vi "Save bline to memory2.vi"(0 "PSOCTSpectral Bline":u16[](array[numeric]), 1 "action":T1=enum."Save(ThorOCT)", 5 "index (row)":i32, 9 "PSOCT Spatial Bline":sgl[](array[numeric]), 11 "error in":errorcluster) -> (15 "error out":errorcluster)   [LabVIEW 2018]
uses:
  Controls/Save Bline to Mem Control.ctl
  Controls/FGV Actions.ctl
  Controls/Queue Manager Actions.ctl
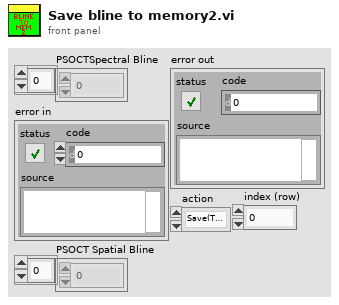
[diagram p1: front panel]
types:
  T1 = typedef "Save Bline to Mem Control.ctl" = enum16{"Output data", "Save(ThorOCT)", "Save(PSOCT)", "FFT and Save", "Uninit", "PSOCT Spectral buffer Set", "PSOCT Spatial buffer Set", "PSOCT Spectral buffer Init", "PSOCT Spatial buffer Init", "ThorOCT Spectral buffer Init", "ThorOCT Spatial buffer Init", "ThorOCT Spectral buffer Set", "ThorOCT Spatial buffer Set", "ThorOCT Spectral Save", "Alazar Spectral Save", "PSOCT save all"}
  T2 = typedef "FGV Actions.ctl" = enum16{"Init", "Set", "Get", "Clear"}
  T3 = typedef "System Parameters.ctl" = cluster{"Optical Parameters":T4, "Vibratome":T5, "Table Stages":T6, "Imaging Parameter":T9, "Galvo HW Parameters":cluster{"Analog Out Channel":tag, "Min Voltage":dbl, "Max Voltage":dbl, "Pixel Clock Source":tag, "Sample Rate":dbl, "Line Clock Out Ch":tag, "2P ready check":tag}, "Alazar parameters":T11, "Mosaic Paramter":cluster{"X Axis":cluster{"Start [mm]":dbl, "Steps [pts]":dbl, "End [mm]":dbl}, "Y Axis":cluster{"Start [mm]":dbl, "Steps [pts]":dbl, "End [mm]":dbl}, "Scan Pattern":enum16{"Uni-directional", "Bi-Directional", "Spiral Out", "Spiral In"}, "Overlap Options":cluster{"Overlap Type":enum16{"No Overlap", "X Only", "Y Only", "X and Y"}, "Percent Overlap":u8, "Justify":enum16{"Start", "Center", "End"}}}, "Manual Controls":T18, "Vibratome Axis":T21}
  T4 = typedef "Optical Parameters.ctl" = cluster{"Obj. Focal Length [mm]":dbl, "Scan Lens EFL[mm]":dbl, "Tube Lens EFL[mm]":dbl, "Galvo V Range (+/-)":dbl, "Galvo Max Half Angle [Deg]":dbl, "Max Galvo Range[%]":dbl}
  T5 = typedef "Vibratome Parameters.ctl" = cluster{"Z Bottom [mm]":dbl, "Pre Cut Dwell [s]":dbl, "Blade Frequency [RPM]":u16, "Slice Speed [mm/s]":dbl, "Post Cut Dwell [s]":dbl, "Ramp Time [s]":dbl, "Start X [mm]":dbl, "Start Y [mm]":dbl, "Slice Length [mm]":dbl, "Slice Axis":enum16{"X Axis", "Y Axis", "Z Axis"}, "Controller VISA Ref":refnum<visa-resource-name>, "Blade Frequency [Hz]":u16, "Analog Out Channel":tag, "Pixel Clock Source":tag}
  T6 = typedef "Translation Stage Parameters.ctl" = cluster{"X Stage":T7, "Y Stage":T7, "Z Stage":T7}
  T7 = typedef "Translation Stage Cluster.ctl" = cluster{"Position":dbl, "Is.Enabled?":bool, "Is.Connected?":bool, "Device SN":string, "AccelerationMaximum":dbl, "VelocityMaximum":dbl, "Acceleration":dbl, "Velocity":dbl, "waitTimeout (ms)":i32, "Model":T8, "Is.Homed?":bool, "MOVE":bool}
  T8 = typedef "Translation Stage Types.ctl" = enum16{"None", "Thorlabs LTS", "Thorlabs MLJ"}
  T9 = typedef "Imaging Parameters.ctl" = cluster{"Raster Scan Direction":T10, "Pixel Dwell Time [Clock Cycles]":u16, "Flyback Time [Clock Cycles]":u16, "XY Center [um]":cluster{"X":dbl, "Y":dbl}, "Pixel Step Size [um] X":dbl, "XY Image Size":enum16{"32 x 32", "64 x 64", "128 x 128", "256 x 256", "512 x 512", "1024 x 1024", "2048 x 2048"}, "Custom":bool, "Custom Size":cluster{"X":u16, "Y":u16}, "Line Averages":u8, "Pixel Step Size [um] Y":dbl}
  T10 = typedef "Scan Direction.ctl" = enum16{"Uni Directional", "Bi Directional", "None"}
  T11 = typedef "Alazar parameters.ctl" = cluster{"Trigger Settings":cluster{"General Trigger Settings":T12, "Trigger Engine 1":T13, "Trigger Engine 2":T13}, "Device ID":T14, "Ch A Input Control":T15, "Ch B Input Control":T15, "Acq Settings":T16, "Capture Clock":T17}
  T12 = typedef "General Trigger Settings.ctl" = cluster{"Trigger Operation":u32, "Coupling ID":u32, "Range ID":u32, "Delay":u32, "Timeout Ticks":u32, "Mode":u32, "Parameter":u32}
  T13 = typedef "Trigger Engine Controls.ctl" = cluster{"Trigger Engine":u32, "Source":u32, "Slope":u32, "Level":u32}
  T14 = typedef "Alazar Device ID.ctl" = cluster{"System ID":u32, "Board ID":u32}
  T15 = typedef "Channel Input Controls.ctl" = cluster{"Channel":u8, "Coupling":u32, "Range":u32, "Impedance":u32}
  T16 = typedef "Alazar Acquisition Settings.ctl" = cluster{"Record Length":u32, "Offset":u32, "Records Per Buffer":u32, "Records Count (Records/Acq)":u32, "Window Type":u32, "Footer":u32, "Samples per record":u32, "Output Format":u32}
  T17 = typedef "Clock Controls.ctl" = cluster{"Sample Rate":u32, "Decimation":u32, "Source":u32, "Edge":u32}
  T18 = typedef "Manual Controls.ctl" = cluster{"Z0":dbl, "First image height":dbl, "Data Path":path, "Save parameters":T19, "Center Galvos":bool, "Acquisition mode":T20, "PSOCT Channel":u32, "Save":bool, "AIP rotation angle":dbl, "ret ds":bool, "Pause?":bool, "Outgoing Mail Server (SMTP)":string, "Email":string, "Password":string, "Carrier 1":enum16{"T-Mobile", "AT&T", "Verizon", "Sprint"}, "phone number 1":string, "Subject":string, "Message":string, "blocker position":enum16{"every two slices", "Nat slices", "None"}, "Carrier 2":enum16{"T-Mobile", "AT&T", "Verizon", "Sprint"}, "phone number 2":string}
  T19 = typedef "FFT parameters.ctl" = cluster{"start pixel":i32, "#pixels to save":i32}
  T20 = typedef "FFT mode.ctl" = enum16{"ThorOCT B line", "ThorOCT Spectral", "ThorOCT FFT", "Alazar B line", "Alazar FFT", "GPU FFT", "Alazar Spectral", "Simulation", "auto adjust focus", "Save all"}
  T21 = typedef "Vibratome Param.ctl" = cluster{"Start [mm](first cut height)":dbl, "slice thickness[um]":dbl, "#slice":u16, "image thickness(um)":dbl, "#images":u16, "30um?":bool}
  T22 = typedef "Queue Manager Actions.ctl" = enum16{"Init", "Enqueue", "Enqueue All", "Preview Queue", "Dequeue", "Get Status", "Flush Queue", "Flush All Queues", "Release All Queues", "Release Queue", "Enqueue at Opposite End"}
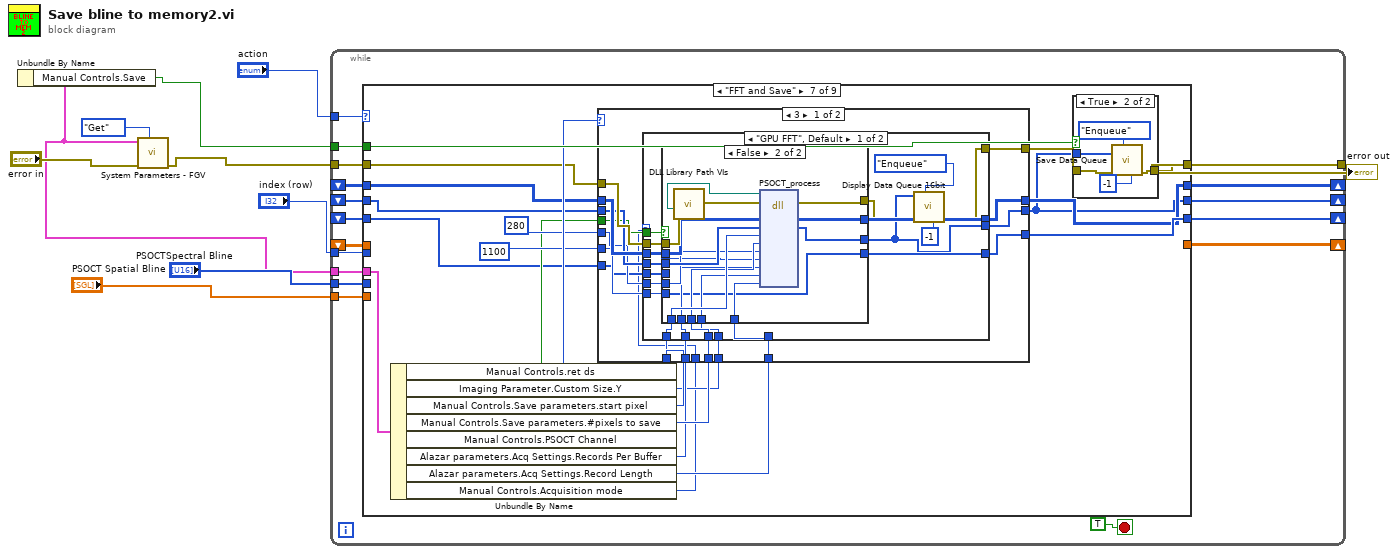
[diagram p0: block diagram]
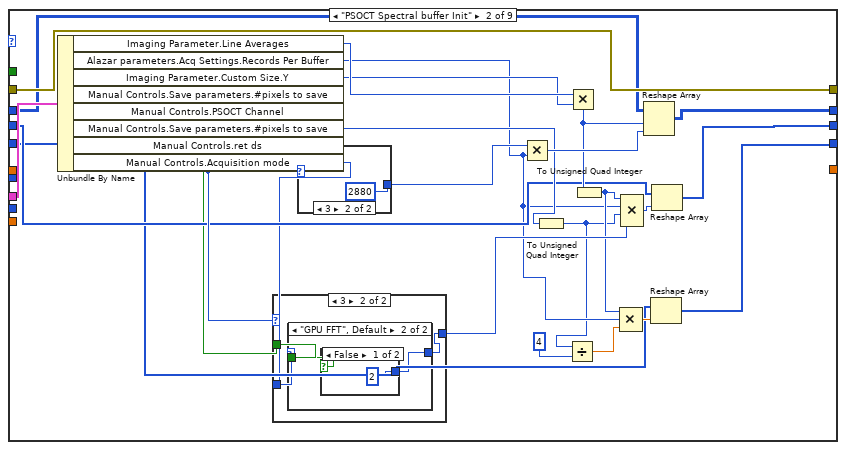
[diagram p3: hidden frame]
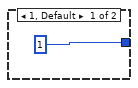
[diagram p4: hidden frame]
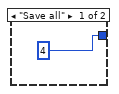
[diagram p5: hidden frame]
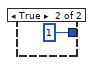
[diagram p6: hidden frame]
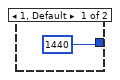
[diagram p7: hidden frame]
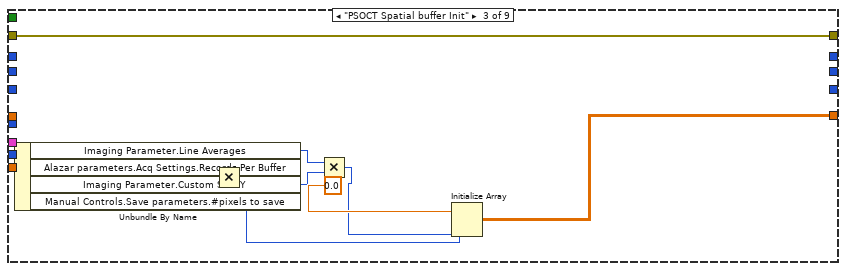
[diagram p8: hidden frame]
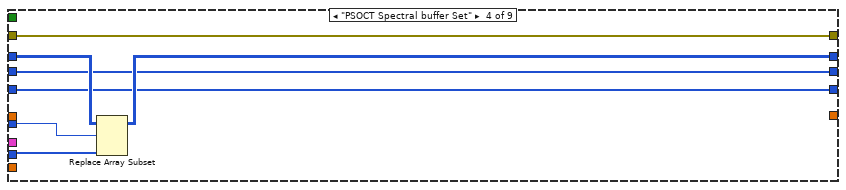
[diagram p9: hidden frame]
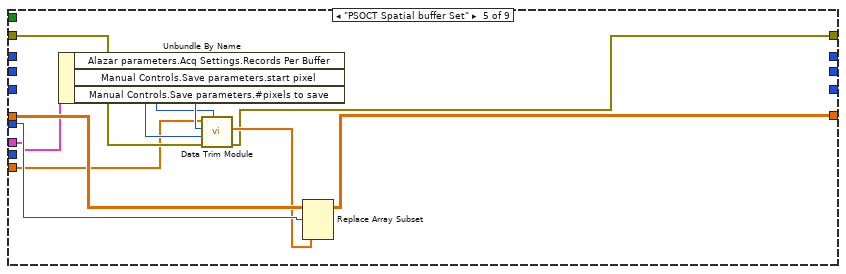
[diagram p10: hidden frame]
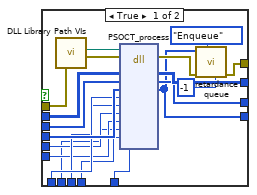
[diagram p12: hidden frame]
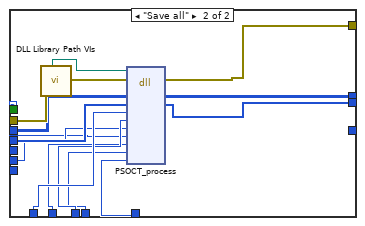
[diagram p13: hidden frame]
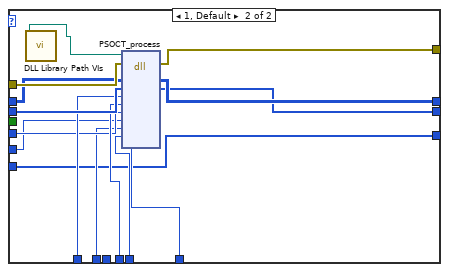
[diagram p14: hidden frame]
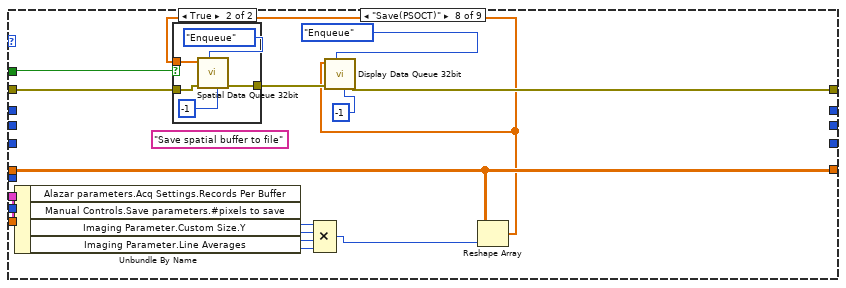
[diagram p16: hidden frame]
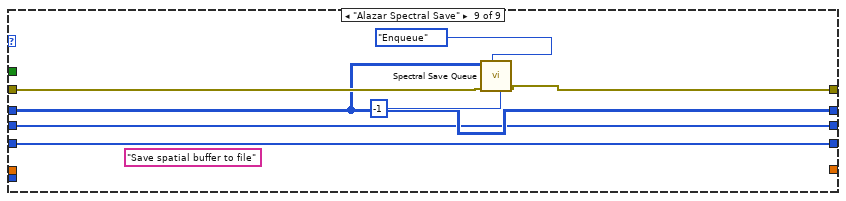
[diagram p18: hidden frame]
diagram:
  n1 = call "System Parameters - FGV.vi"("Actions"=FGV_Actions."Get", "Error In"="error in") -> ("Error Out"=w3:errorcluster, "System Parameters [Out]"=w2:T3)  [unwired: 8 in]
  n2 = Unbundle By Name(w2) -> ("Manual Controls.Save"=w1:bool)
  n3 = while {
    tunnel: "action" -> [w27]
    shift-right: [w26] -> _
    shift-left: _ -> [w25]
    tunnel: "PSOCTSpectral Bline" -> [w24]
    tunnel: "index (row)" -> [w22]
    tunnel: w3 -> [w21]
    tunnel: w2 -> [w20]
    tunnel: [w19] -> w6
    shift-right: [w18] -> _
    shift-left: _ -> [w17]
    tunnel: "PSOCT Spatial Bline" -> [w16]
    tunnel: w1 -> [w15]
    shift-right: [w14] -> _
    shift-left: _ -> [w13]
    shift-right: [w12] -> _
    shift-left: _ -> [w11]
    stop <- TRUE stop-if-true
    n4 = case shown="\"FFT and Save\"" w27 {
      tunnel: [w32 w56 _ w82 _ _ w100 _ w246] -> w26
      tunnel: w25 -> [w32 w44 _ w85 _ _ w114 _ w246]
      tunnel: w24 -> [_ _ _ w83 _ _ _ _ _]
      tunnel: w22 -> [_ _ _ w84 w94 _ _ _ _]
      tunnel: w21 -> [w30 w52 w69 w81 w90 w97 w115 w237 w249]
      tunnel: w20 -> [_ w55 w76 _ w91 _ w118 w235 _]
      tunnel: [w30 w52 w69 w81 w86 w97 w99 w225 w248] -> w19
      tunnel: [w31 _ w73 _ w95 _ _ w236 _] -> w18
      tunnel: w17 -> [w31 _ _ _ w96 _ _ w236 _]
      tunnel: w16 -> [_ _ _ _ w88 _ _ _ _]
      tunnel: w15 -> [_ _ _ _ _ _ w117 w227 _]
      tunnel: [w29 w49 _ w80 _ _ w98 _ w245] -> w14
      tunnel: w13 -> [w29 w43 _ w80 _ _ w113 _ w245]
      tunnel: [w28 w36 _ w79 _ _ w103 _ w244] -> w12
      tunnel: w11 -> [w28 w35 _ w79 _ _ w102 _ w244]
      frame Default {
      }
      frame "PSOCT Spectral buffer Init" {
        n5 = Unbundle By Name(w55) -> ("Imaging Parameter.Line Averages"=w54:u8, "Alazar parameters.Acq Settings.Records Per Buffer"=w40:u32, "Imaging Parameter.Custom Size.Y"=w53:u16, "Manual Controls.PSOCT Channel"=w50:u32, "Manual Controls.Save parameters.#pixels to save"=w48:i32, "Manual Controls.ret ds"=w34:bool, "Manual Controls.Acquisition mode"=w33:T20)  [unwired: 1 out]
        n6 = case shown="3" w50 {
          tunnel: [u64 1 ("element") w61] -> w45
          tunnel: w34 -> [_ w60]
          tunnel: w33 -> [_ w59]
          frame 1, Default {
          }
          frame 3 {
            n7 = case shown="\"GPU FFT\", Default" w59 {
              tunnel: [4 w64] -> w61
              tunnel: w60 -> [_ w63]
              frame "Save all" {
              }
              frame "GPU FFT", Default {
                n8 = case shown="False" w63 {
                  tunnel: [2 u64 1 ("element")] -> w64
                  frame False {
                  }
                  frame True {
                  }
                }
              }
            }
          }
        }
        n9 = case shown="3" w50 {
          tunnel: [u32 1440 ("element") u32 2880 ("element")] -> w51
          frame 1, Default {
          }
          frame 3 {
          }
        }
        n10 = Multiply(x=w51, y=w40) -> (x*y=w57:u32)
        n11 = To Unsigned Quad Integer(1:w48) -> (0:w38:u64)
        n12 = Divide(x=w38, y=u64 4) -> (x/y=w39:dbl)
        n13 = Multiply(x=w54, y=w53) -> (x*y=w47:u16)
        n14 = To Unsigned Quad Integer(1:w47) -> (0:w41:u64)
        n15 = Compound Arithmetic op=MULTIPLY(w41, w40, w39) -> (w42:dbl)
        n16 = Compound Arithmetic op=MULTIPLY(w41, w40, w38, w45) -> (w46:u64)
        n17 = Reshape Array(w44, w47, w57) -> (w56:u16[][])
        n18 = Reshape Array(w35, w42) -> (w36:u16[])
        n19 = Reshape Array(w43, w46) -> (w49:u16[])
      }
      frame "PSOCT Spatial buffer Init" {
        n20 = Unbundle By Name(w76) -> ("Imaging Parameter.Line Averages"=w72:u8, "Alazar parameters.Acq Settings.Records Per Buffer"=w74:u32, "Imaging Parameter.Custom Size.Y"=w71:u16, "Manual Controls.Save parameters.#pixels to save"=w75:i32)
        n21 = Multiply(x=w74, y=w75) -> (x*y=w77:u32)
        n22 = Multiply(x=w72, y=w71) -> (x*y=w70:u16)
        n23 = Initialize Array(sgl 0.0 ("element"), w70, w77) -> (w73:sgl[][])
      }
      frame "PSOCT Spectral buffer Set" {
        n24 = Replace Array Subset(array=w85, new element=w83, index (row)=w84) -> (w82:u16[][])  [unwired: 1 in]
      }
      frame "PSOCT Spatial buffer Set" {
        n25 = Unbundle By Name(w91) -> ("Alazar parameters.Acq Settings.Records Per Buffer"=w93:u32, "Manual Controls.Save parameters.start pixel"=w92:i32, "Manual Controls.Save parameters.#pixels to save"=w87:i32)
        n26 = call "Data Trim Module.vi"("#pixels to save"=w87, "error in"=w90, "start pixel"=w92, "#A-lines"=w93, "1D Array in"=w88) -> ("error out"=w86:errorcluster, "array for saving"=w89:sgl[])  [unwired: 5 in]
        n27 = Replace Array Subset(array=w96, new element=w89, index (row)=w94) -> (w95:sgl[][])  [unwired: 1 in]
      }
      frame "Uninit" {
      }
      frame "FFT and Save" {
        n28 = Unbundle By Name(w118) -> ("Manual Controls.ret ds"=w104:bool, "Imaging Parameter.Custom Size.Y"=w107:u16, "Manual Controls.Save parameters.start pixel"=w112:i32, "Manual Controls.Save parameters.#pixels to save"=w111:i32, "Manual Controls.PSOCT Channel"=w116:u32, "Alazar parameters.Acq Settings.Records Per Buffer"=w108:u32, "Alazar parameters.Acq Settings.Record Length"=w106:u32, "Manual Controls.Acquisition mode"=w101:T20)
        n29 = case shown="3" w116 {
          tunnel: w115 -> [w135 w215]
          tunnel: w114 -> [w134 w214]
          tunnel: w113 -> [w133 w213]
          tunnel: w112 -> [w132 w212]
          tunnel: w111 -> [w131 w211]
          tunnel: i16 280 ("a") -> [w130 w210]
          tunnel: i16 1100 ("b") -> [w129 w209]
          tunnel: w108 -> [w128 w208]
          tunnel: w107 -> [w127 w207]
          tunnel: w106 -> [w126 w206]
          tunnel: [w125 w216] -> w105
          tunnel: [w124 w205] -> w100
          tunnel: [w123 w204] -> w98
          tunnel: w104 -> [w122 _]
          tunnel: [w121 w203] -> w103
          tunnel: w102 -> [w120 w203]
          tunnel: w101 -> [w119 _]
          frame 3 {
            n30 = case shown="\"GPU FFT\", Default" w119 {
              tunnel: w135 -> [w154 w202]
              tunnel: w134 -> [w153 w201]
              tunnel: w133 -> [w152 w200]
              tunnel: w132 -> [w151 w199]
              tunnel: w131 -> [w150 w198]
              tunnel: w130 -> [w149 w197]
              tunnel: w129 -> [w148 w196]
              tunnel: w128 -> [w147 w195]
              tunnel: w127 -> [w146 w194]
              tunnel: w126 -> [w145 w193]
              tunnel: [w137 w192] -> w125
              tunnel: [w144 w191] -> w124
              tunnel: [w136 w190] -> w123
              tunnel: w122 -> [w143 _]
              tunnel: [w142 _] -> w121
              tunnel: w120 -> [w141 _]
              frame "GPU FFT", Default {
                n31 = case shown="False" w143 {
                  tunnel: w154 -> [w172 w187]
                  tunnel: w153 -> [w169 w186]
                  tunnel: w152 -> [w168 w185]
                  tunnel: w151 -> [w166 w184]
                  tunnel: w150 -> [w165 w183]
                  tunnel: w149 -> [w164 w182]
                  tunnel: w148 -> [w163 w181]
                  tunnel: w147 -> [w162 w180]
                  tunnel: w146 -> [w161 w179]
                  tunnel: w145 -> [w160 w178]
                  tunnel: [w158 w177] -> w138
                  tunnel: [w171 w176] -> w144
                  tunnel: [w170 w175] -> w136
                  tunnel: [w157 w174] -> w142
                  tunnel: w141 -> [w167 w174]
                  frame True {
                    n32 = call "DLL Library Path VIs.vi"() -> ("GPU FFT birefringence simple ret"=w173:path)  [unwired: 5 in, 6 out]
                    n33 = dll-call lib="C:/Project/SerialSectionOCT/SerialSectOCT/Labview Software/DLL/CUDA_FFT_2_channel_ref_ret_fast2.dll" fn="PSOCT_process"(path in=w173, error in=w172, "h_signal"=w169, "h_processed_ref"=w168, "h_processed_ret"=w167, "Z0"=w166, "DEPTH"=w165, "a"=w164, "b"=w163, "NALINES"=w162, "NBLINES"=w161, "SAMPLES"=w160) -> (error out=w159:errorcluster, "h_signal"=w171:u16[][], "h_processed_ref"=w170:u16[], "h_processed_ret"=w157:u16[])  [unwired: 9 in, 1 out]
                    n34 = call "retardance queue.vi"("timeout in ms (-1)"=-1, "Action"=Queue_Manager_Actions."Enqueue", "error in (no error)"=w159, "data in"=w157) -> ("error out"=w158:errorcluster)  [unwired: 4 in, 3 out]
                  }
                  frame False {
                    n35 = call "DLL Library Path VIs.vi"() -> ("GPU FFT amps"=w188:path)  [unwired: 5 in, 6 out]
                    n36 = dll-call lib="C:/Project/SerialSectionOCT/SerialSectOCT/Labview Software/DLL/CUDA_FFT_2_channel_amps.dll" fn="PSOCT_process"(path in=w188, error in=w187, "h_signal"=w186, "h_processed_amps"=w185, "Z0"=w184, "DEPTH"=w183, "a"=w182, "b"=w181, "NALINES"=w180, "NBLINES"=w179, "SAMPLES"=w178) -> (error out=w177:errorcluster, "h_signal"=w176:u16[][], "h_processed_amps"=w175:u16[])  [unwired: 9 in, 1 out]
                  }
                }
                n37 = call "Display Data Queue 16bit.vi"("timeout in ms (-1)"=-1, "Action"=Queue_Manager_Actions."Enqueue", "error in (no error)"=w138, "data in"=w136) -> ("error out"=w137:errorcluster)  [unwired: 4 in, 3 out]
              }
              frame "Save all" {
                n38 = call "DLL Library Path VIs.vi"() -> ("GPU FFT Save all"=w189:path)  [unwired: 5 in, 6 out]
                n39 = dll-call lib="C:/Project/SerialSectionOCT/SerialSectOCT/Labview Software/DLL/CUDA_FFT_2_channel_save_all.dll" fn="PSOCT_process"(path in=w189, error in=w202, "h_signal"=w201, "h_processed_save_all"=w200, "Z0"=w199, "DEPTH"=w198, "a"=w197, "b"=w196, "NALINES"=w195, "NBLINES"=w194, "SAMPLES"=w193) -> (error out=w192:errorcluster, "h_signal"=w191:u16[][], "h_processed_save_all"=w190:u16[])  [unwired: 9 in, 1 out]
              }
            }
          }
          frame 1, Default {
            n40 = call "DLL Library Path VIs.vi"() -> ("GPU FFT amplitude"=w217:path)  [unwired: 5 in, 6 out]
            n41 = dll-call lib="C:/Project/SerialSectionOCT/SerialSectOCT/Labview Software/DLL/CUDA_FFT_single_channel.dll" fn="PSOCT_process"(path in=w217, error in=w215, "h_signal"=w214, "h_processed_signal"=w213, "Z0"=w212, "DEPTH"=w211, "a"=w210, "b"=w209, "NALINES"=w208, "NBLINES"=w207, "SAMPLES"=w206) -> (error out=w216:errorcluster, "h_signal"=w205:u16[][], "h_processed_signal"=w204:u16[])  [unwired: 9 in, 1 out]
          }
        }
        n42 = case shown="True" w117 {
          tunnel: w105 -> [w218 w223]
          tunnel: [w218 w222] -> w99
          tunnel: w98 -> [_ w219]
          frame False {
          }
          frame True {
            n43 = call "Save Data Queue.vi"("timeout in ms (-1)"=-1, "Action"=Queue_Manager_Actions."Enqueue", "error in (no error)"=w223, "data in"=w219) -> ("error out"=w222:errorcluster)  [unwired: 4 in, 3 out]
          }
        }
      }
      frame "Save(PSOCT)" {
        (unwired) "Save spatial buffer to file"
        n44 = Unbundle By Name(w235) -> ("Alazar parameters.Acq Settings.Records Per Buffer"=w234:u32, "Manual Controls.Save parameters.#pixels to save"=w233:i32, "Imaging Parameter.Custom Size.Y"=w232:u16, "Imaging Parameter.Line Averages"=w226:u8)
        n45 = Compound Arithmetic op=MULTIPLY(w234, w233, w232, w226) -> (w231:u32)
        n46 = Reshape Array(w236, w231) -> (w224:sgl[])
        n47 = case shown="True" w227 {
          tunnel: w237 -> [w238 w243]
          tunnel: [w238 w242] -> w230
          tunnel: w224 -> [_ w239]
          frame False {
          }
          frame True {
            n48 = call "Spatial Data Queue 32bit.vi"("timeout in ms (-1)"=-1, "Action"=Queue_Manager_Actions."Enqueue", "error in (no error)"=w243, "data in"=w239) -> ("error out"=w242:errorcluster)  [unwired: 4 in, 3 out]
          }
        }
        n49 = call "Display Data Queue 32bit.vi"("timeout in ms (-1)"=-1, "Action"=Queue_Manager_Actions."Enqueue", "error in (no error)"=w230, "data in"=w224) -> ("error out"=w225:errorcluster)  [unwired: 4 in, 3 out]
      }
      frame "Alazar Spectral Save" {
        (unwired) "Save spatial buffer to file"
        n50 = call "Spectral Save Queue.vi"("timeout in ms (-1)"=-1, "Action"=Queue_Manager_Actions."Enqueue", "error in (no error)"=w249, "data in"=w246) -> ("error out"=w248:errorcluster)  [unwired: 4 in, 3 out]
      }
    }
  }
  "error out" <- w6
